vi "Get cif_management_common_TimingStatistics.vi"(8 "error in (no error)":errorcluster, 11 "gRPCid":T1) -> (0 "error out":errorcluster, 2 "package_templatemessage":T2, 3 "gRPCid out":T1)   [LabVIEW 2021, in "CIF_PluginLoader_server.lvlib"]
uses:
  CIF_PluginLoader_server.lvlib
  cif_management_common_TimingStatistics.ctl
  cif_common_TimingStats.ctl
  <vilib>/gRPC/LabVIEW gRPC Library/Shared/grpcId.ctl
  cif_management_common_TimingStatistics_Flat.ctl
  cif_common_TimingStats_Flat.ctl
  2ed25e12-861d-4677-8ead-ace2906b2041.vi
  <vilib>/gRPC/LabVIEW gRPC Library/Shared/TranslateGrpcError.vi
  FlatToRichcif_common_TimingStats.vi
  <vilib>/gRPC/LabVIEW gRPC Library/Server API/Server/Get Server DLL Path.vi
  <vilib>/Utility/error.llb/Error Cluster From Error Code.vi
  <vilib>/gRPC/LabVIEW gRPC Library/grpc-lvsupport-release.lvlib
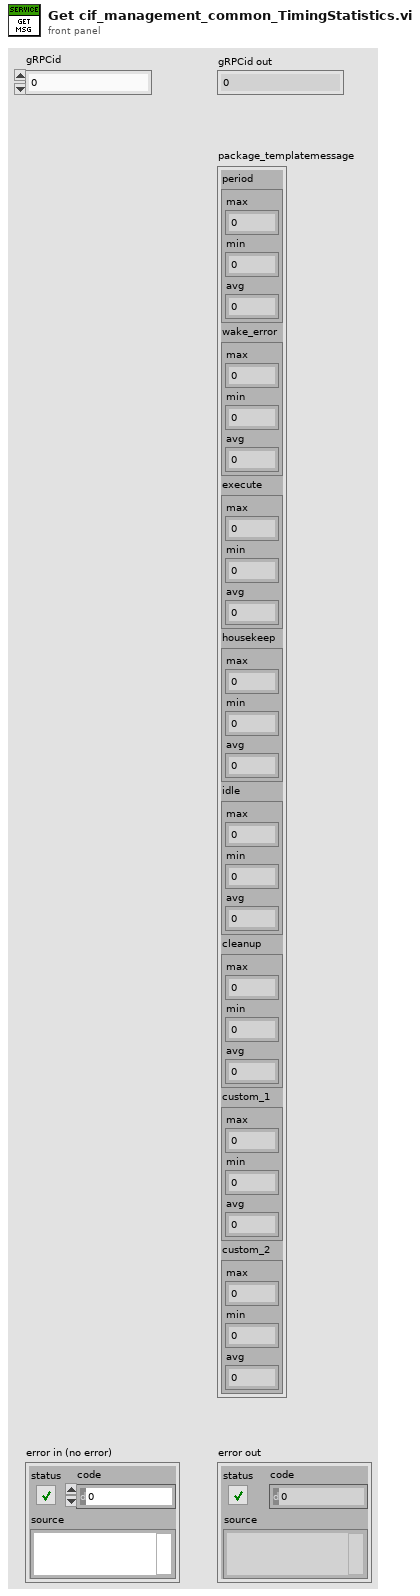
[diagram p1: front panel]
types:
  T1 = typedef "grpc-lvsupport-release.lvlib/grpcId.ctl" = u64
  T2 = typedef "CIF_PluginLoader_server.lvlib/cif_management_common_TimingStatistics.ctl" = cluster{"period":T3, "wake_error":T3, "execute":T3, "housekeep":T3, "idle":T3, "cleanup":T3, "custom_1":T3, "custom_2":T3}
  T3 = typedef "CIF_PluginLoader_server.lvlib/cif_common_TimingStats.ctl" = cluster{"max":i64, "min":i64, "avg":dbl}
  T4 = typedef "CIF_PluginLoader_server.lvlib/cif_management_common_TimingStatistics_Flat.ctl" = cluster{"period":T5, "wake_error":T5, "execute":T5, "housekeep":T5, "idle":T5, "cleanup":T5, "custom_1":T5, "custom_2":T5}
  T5 = typedef "CIF_PluginLoader_server.lvlib/cif_common_TimingStats_Flat.ctl" = cluster{"max":i64, "min":i64, "avg":dbl}
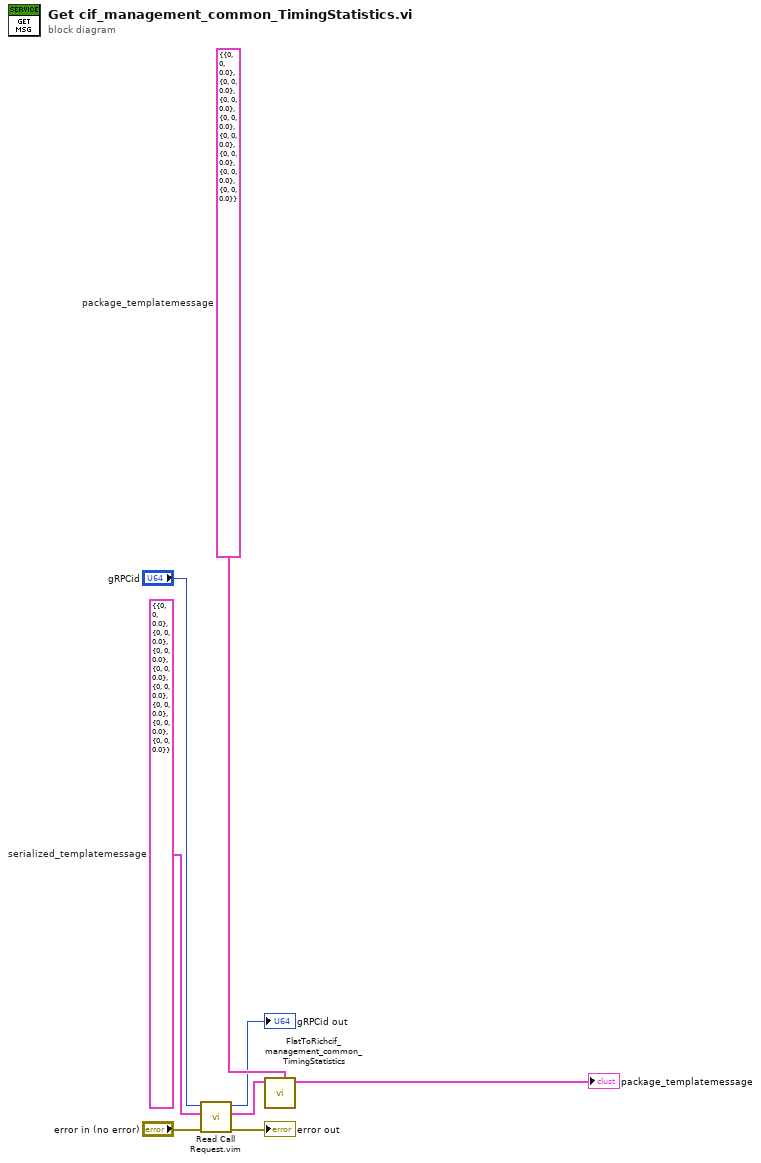
[diagram p0: block diagram]
diagram:
  w6 = T4 {"period"={"max"=0, "min"=0, "avg"=0.0}, "wake_error"={"max"=0, "min"=0, "avg"=0.0}, "execute"={"max"=0, "min"=0, "avg"=0.0}, "housekeep"={"max"=0, "min"=0, "avg"=0.0}, "idle"={"max"=0, "min"=0, "avg"=0.0}, "cleanup"={"max"=0, "min"=0, "avg"=0.0}, "custom_1"={"max"=0, "min"=0, "avg"=0.0}, "custom_2"={"max"=0, "min"=0, "avg"=0.0}}  # serialized_templatemessage
  w5 = T2 {"period"={"max"=0, "min"=0, "avg"=0.0}, "wake_error"={"max"=0, "min"=0, "avg"=0.0}, "execute"={"max"=0, "min"=0, "avg"=0.0}, "housekeep"={"max"=0, "min"=0, "avg"=0.0}, "idle"={"max"=0, "min"=0, "avg"=0.0}, "cleanup"={"max"=0, "min"=0, "avg"=0.0}, "custom_1"={"max"=0, "min"=0, "avg"=0.0}, "custom_2"={"max"=0, "min"=0, "avg"=0.0}}  # package_templatemessage
  n1 = call "Read Call Request.vim"("error in"="error in (no error)", "Request Type"=w6, "gRPCid in"="gRPCid") -> ("error out"=→"error out":errorcluster, "Request Data"=w4:T4, "gRPCid out"=→"gRPCid out":T1)  [unwired: 6 in]
  n2 = call "FlatToRichcif_management_common_TimingStatistics.vi"("OutputClusterType"=w5, "InputCluster"=w4) -> ("OutputCluster"=→"package_templatemessage":T2)  [unwired: 9 in]
